vi "SaveDeviceHeader.vi"(0 "File Refnum in":refnum<file>, 1 "no. of arrays":i32, 3 "Array Lengths":i32, 5 "Filename":string, 7 "Run Number":i32, 9 "Array Titles":string, 11 "error in (no error)":errorcluster, 12 "Temperature":dbl, 13 "Humidity":dbl, 14 "Strip Segment":string) -> (4 "File Refnum out":refnum<file>, 6 "Header string":string, 10 "error out":errorcluster)   [LabVIEW 2013]
uses:
  globals/QC_RunInformation.vi
  globals/QC_MeasurementSetup.vi
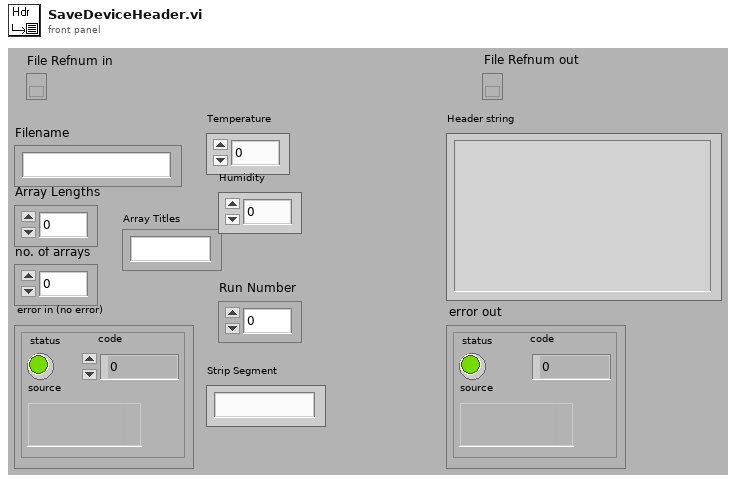
[diagram p1: front panel]
types:
  T1 = cluster{"Institute":string, "Manufacturers":string[], "Devices":string[], "Serialnumbers Lookup DB":string, "Data directory":string, "Backup & screenshot directory":string, "List of known users":string[], "Measurement switch not used":bool, "Measurement Switch":string, "DUT Switch":string, "Rseries IV [MOhm]":string, "Rshunt IV [MOhm]":string, "Rseries CV [MOhm]":string, "DC blocking Cap [µF]":string, "Rseries LCR [MOhm]":string, "Rseries stability [MOhm]":string, "Rshunt stability [MOhm]":string, "Rseries striptest bias [MOhm]":string, "Rseries strip pinhole [MOhm]":string}
  T2 = cluster{"Sensor Serial No.:":string, "Wafer:":string, "Batch:":string, "Manufacturer:":string, "Device Category:":string, "Database Serial No.:":string, "Date Initiated:":string, "Time Initiated:":string, "Test":string, "Probeplan used:":string, "End of Run comment:":string, "User:":string, "Vbias SMU":string, "LCR":string, "Test SMU":string, "Test DMM":string}
  T3 = cluster{"Supply":refnum<class "SupplyControl.lvclass">, "LCR":refnum<class "LCRControl.lvclass">, "Initial Voltage [V]":dbl, "Final Voltage [V]":dbl, "Step Size [V]":dbl, "Step Interval [s]":i32, "Number Of Steps":u32, "AC frequency [Hz]":i32, "RC Configuration":u16, "AC amplitude [V]":dbl, "Ramp down steps [V]":dbl, "Ramp down Interval [s]":i32, "Set Current Limit?":bool, "Current Limit [µA]":dbl, "Temperature Readout":enum16{"Read Arduino", "Enter manually"}, "Arduino":refnum<class "ArduinoControl.lvclass">, "Supply Name":string, "LCR Name":string, "V_depletion Limit [V]":dbl, "Switching":refnum<class "Switching.lvclass">, "Matrix used?":bool, "Matrix X Channels":cluster{"Bias Supply / SMU LO":i32, "Bias Supply / SMU HI":i32, "CV Box LO":i32, "CV Box HI":i32, "CV Box LO IN":i32, "CV Box HI IN":i32, "Volt meter LO":i32, "Volt meter HI":i32, "Mux1 C1":i32, "Mux1 C2":i32, "Mux2 C1":i32, "Mux2 C2":i32}}
  T4 = cluster{"Bias Supply":refnum<class "SupplyControl.lvclass">, "SMU":refnum<class "SupplyControl.lvclass">, "LCR":refnum<class "LCRControl.lvclass">, "Probe Card Channels":i32, "Bias Voltage [V]":dbl, "First strip":i32, "Last strip":i32, "Base Voltage [V]":dbl, "Base Ramp Step [V]":dbl, "Base Ramp Interval [ms]":u32, "High Voltage [V]":dbl, "High Ramp Step [V]":dbl, "High Ramp Interval [ms]":u32, "AC frequency [Hz]":i32, "AC amplitude [V]":dbl, "RC Configuration":u16, "Single Needle":bool, "Temperature Readout":enum16{"Read Arduino", "Enter manually"}, "Arduino":refnum<class "ArduinoControl.lvclass">, "Fraction of good strips [%]":dbl, "ProbeStation":refnum<class "ProbeStationControl.lvclass">, "Switching":refnum<class "Switching.lvclass">, "Matrix used?":bool, "Matrix X Channels":cluster{"Bias Supply / SMU LO":i32, "Bias Supply / SMU HI":i32, "CV Box LO":i32, "CV Box HI":i32, "CV Box LO IN":i32, "CV Box HI IN":i32, "Volt meter LO":i32, "Volt meter HI":i32, "Mux1 C1":i32, "Mux1 C2":i32, "Mux2 C1":i32, "Mux2 C2":i32}, "Pinholes Y/N":bool, "Capacitance Y/N":bool, "Resistance Y/N":bool, "Bias Supply Name":string, "SMU Name":string, "LCR Name":string}
  T5 = cluster{"Supply":refnum<class "SupplyControl.lvclass">, "LCR":refnum<class "LCRControl.lvclass">, "Initial Voltage [V]":dbl, "Final Voltage [V]":dbl, "Step Size [V]":dbl, "Step Interval [s]":i32, "Number Of Steps":u32, "AC frequency [Hz]":i32, "RC Configuration":u16, "AC amplitude [V]":dbl, "Ramp down steps [V]":dbl, "Ramp down Interval [s]":i32, "Set Current Limit?":bool, "Current Limit [µA]":dbl, "Temperature Readout":enum16{"Read Arduino", "Enter manually"}, "Arduino":refnum<class "ArduinoControl.lvclass">, "Supply Name":string, "LCR Name":string, "C_is Limit [pF/cm]":dbl, "Switching":refnum<class "Switching.lvclass">, "Matrix used?":bool, "Matrix X Channels":cluster{"Bias Supply / SMU LO":i32, "Bias Supply / SMU HI":i32, "CV Box LO":i32, "CV Box HI":i32, "CV Box LO IN":i32, "CV Box HI IN":i32, "Volt meter LO":i32, "Volt meter HI":i32, "Mux1 C1":i32, "Mux1 C2":i32, "Mux2 C1":i32, "Mux2 C2":i32}}
  T6 = cluster{"Supply":refnum<class "SupplyControl.lvclass">, "Voltage [V]":dbl, "Measurement Interval [s]":i32, "Test Duration":u32, "Ramp up steps [V]":dbl, "Ramp up Interval [s]":u32, "Ramp down steps [V]":dbl, "Ramp down Interval [s]":i32, "Set Current Limit?":bool, "Current Limit [µA]":dbl, "Temperature Readout":enum16{"Read Arduino", "Enter manually"}, "Arduino":refnum<class "ArduinoControl.lvclass">, "Supply Name":string, "Maximum current fluctuation [%]":dbl, "Switching.lvclass":refnum<class "Switching.lvclass">, "Matrix used?":bool, "Matrix X Channels":cluster{"Bias Supply / SMU LO":i32, "Bias Supply / SMU HI":i32, "CV Box LO":i32, "CV Box HI":i32, "CV Box LO IN":i32, "CV Box HI IN":i32, "Volt meter LO":i32, "Volt meter HI":i32, "Mux1 C1":i32, "Mux1 C2":i32, "Mux2 C1":i32, "Mux2 C2":i32}}
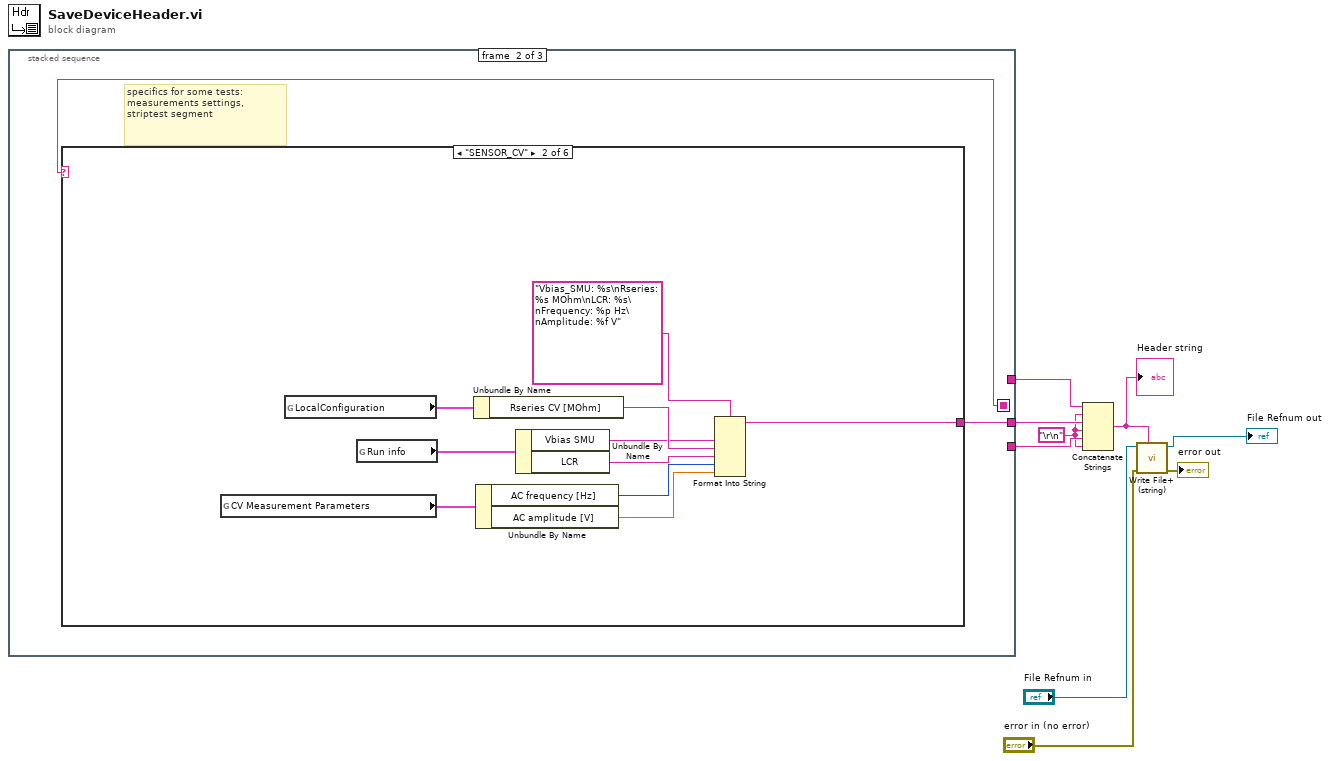
[diagram p0: block diagram]
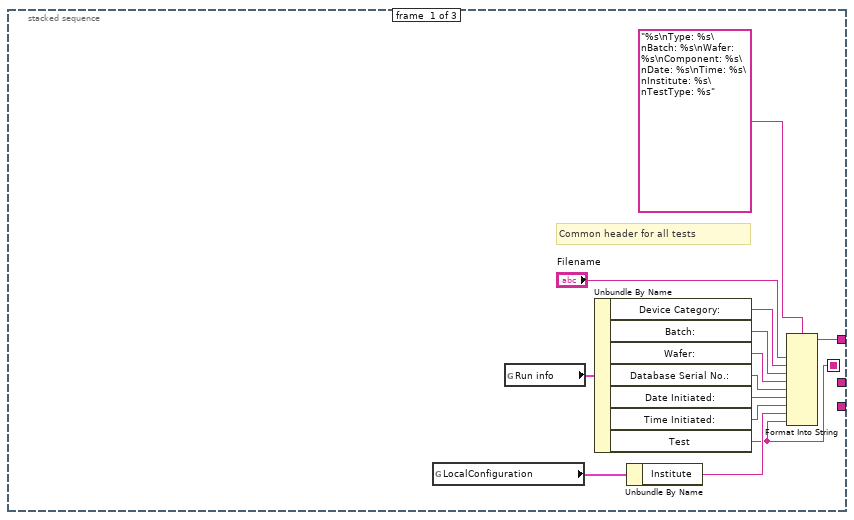
[diagram p2: hidden frame]
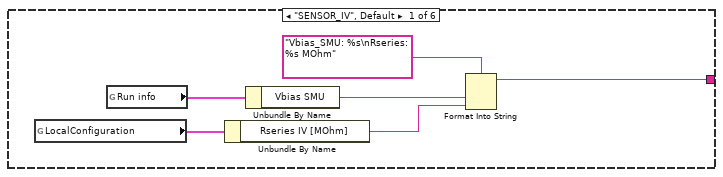
[diagram p3: hidden frame]
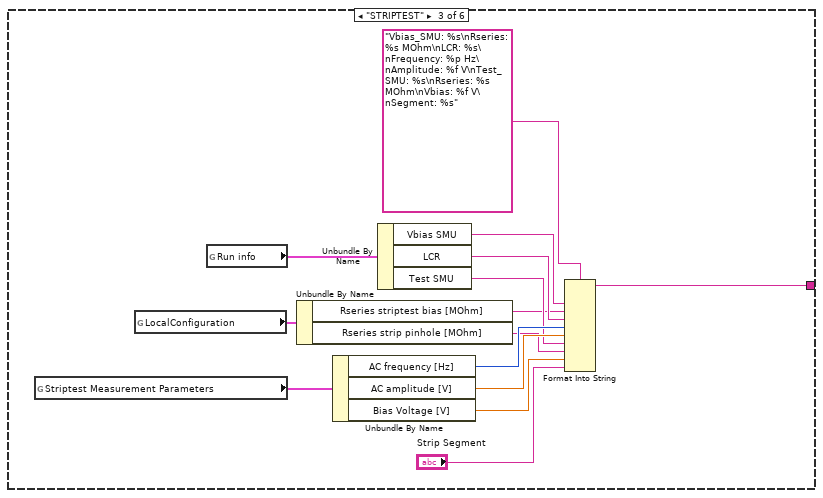
[diagram p4: hidden frame]
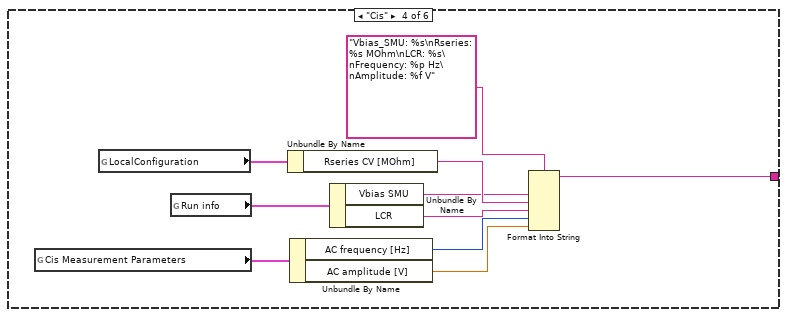
[diagram p5: hidden frame]
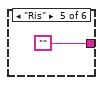
[diagram p6: hidden frame]
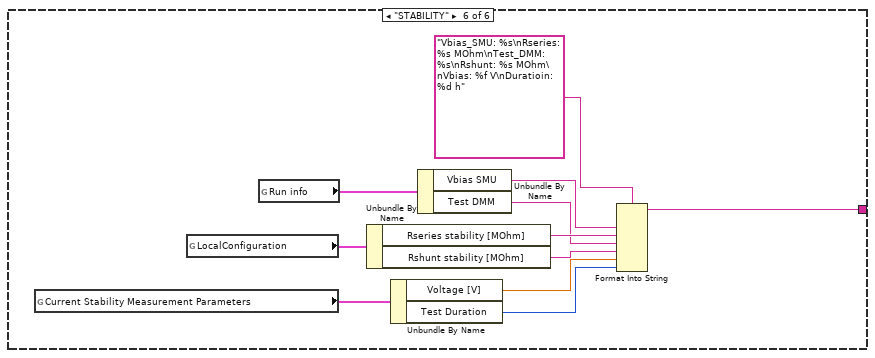
[diagram p7: hidden frame]
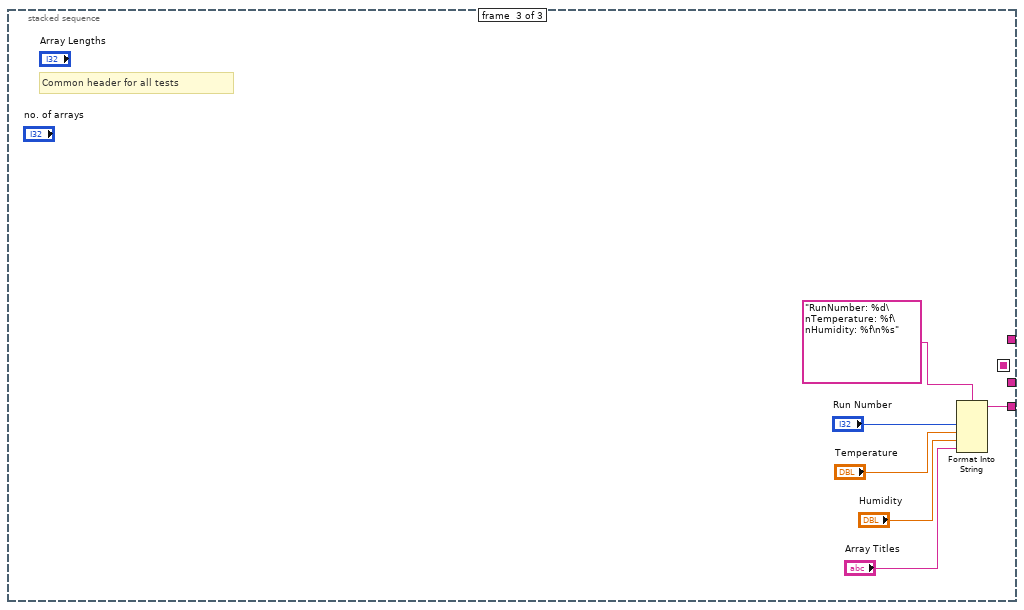
[diagram p8: hidden frame]
diagram:
  w1 = "\r\n"
  n1 = stacked-sequence {
    seq-local: [w11 _ _] -> [_ w24 _]
    tunnel: [_ w23 _] -> w5
    tunnel: [_ _ w77] -> w4
    tunnel: [w10 _ _] -> w3
    frame #0 {
      # "Common header for all tests"
      n2 = global read "QC_RunInformation.vi" "LocalConfiguration"() -> (w12:T1)
      n3 = global read "QC_RunInformation.vi" "Run info"() -> (w13:T2)
      n4 = Unbundle By Name(w13) -> ("Device Category:"=w16:string, "Batch:"=w17:string, "Wafer:"=w18:string, "Database Serial No.:"=w19:string, "Date Initiated:"=w20:string, "Time Initiated:"=w21:string, "Test"=w11:string)
      n5 = Unbundle By Name(w12) -> ("Institute"=w22:string)
      n6 = Format Into String(format string="%s\nType: %s\nBatch: %s\nWafer: %s\nComponent: %s\nDate: %s\nTime: %s\nInstitute: %s\nTestType: %s", "Filename", w16, w17, w18, w19, w20, w21, w22, w11) -> (resulting string=w10:string)  [unwired: 2 in, 1 out]
    }
    frame #1 {
      # "specifics for some tests:\nmeasurements settings,\nstriptest segment"
      n7 = case shown="\"SENSOR_CV\"" w24 {
        tunnel: [w25 w31 w51 w55 "" w72] -> w23
        frame "SENSOR_IV", Default {
          n8 = global read "QC_RunInformation.vi" "LocalConfiguration"() -> (w30:T1)
          n9 = global read "QC_RunInformation.vi" "Run info"() -> (w29:T2)
          n10 = Unbundle By Name(w30) -> ("Rseries IV [MOhm]"=w27:string)
          n11 = Unbundle By Name(w29) -> ("Vbias SMU"=w26:string)
          n12 = Format Into String(format string="Vbias_SMU: %s\nRseries: %s MOhm", w26, w27) -> (resulting string=w25:string)  [unwired: 2 in, 1 out]
        }
        frame "SENSOR_CV" {
          n13 = global read "QC_MeasurementSetup.vi" "CV Measurement Parameters"() -> (w40:T3)
          n14 = global read "QC_RunInformation.vi" "LocalConfiguration"() -> (w39:T1)
          n15 = global read "QC_RunInformation.vi" "Run info"() -> (w38:T2)
          n16 = Unbundle By Name(w39) -> ("Rseries CV [MOhm]"=w36:string)
          n17 = Unbundle By Name(w40) -> ("AC frequency [Hz]"=w33:i32, "AC amplitude [V]"=w32:dbl)
          n18 = Unbundle By Name(w38) -> ("Vbias SMU"=w35:string, "LCR"=w34:string)
          n19 = Format Into String(format string="Vbias_SMU: %s\nRseries: %s MOhm\nLCR: %s\nFrequency: %p Hz\nAmplitude: %f V", w35, w36, w34, w33, w32) -> (resulting string=w31:string)  [unwired: 2 in, 1 out]
        }
        frame "STRIPTEST" {
          n20 = global read "QC_MeasurementSetup.vi" "Striptest Measurement Parameters"() -> (w53:T4)
          n21 = global read "QC_RunInformation.vi" "LocalConfiguration"() -> (w44:T1)
          n22 = global read "QC_RunInformation.vi" "Run info"() -> (w54:T2)
          n23 = Unbundle By Name(w44) -> ("Rseries striptest bias [MOhm]"=w43:string, "Rseries strip pinhole [MOhm]"=w41:string)
          n24 = Unbundle By Name(w53) -> ("AC frequency [Hz]"=w50:i32, "AC amplitude [V]"=w49:dbl, "Bias Voltage [V]"=w42:dbl)
          n25 = Unbundle By Name(w54) -> ("Vbias SMU"=w47:string, "LCR"=w46:string, "Test SMU"=w45:string)
          n26 = Format Into String(format string="Vbias_SMU: %s\nRseries: %s MOhm\nLCR: %s\nFrequency: %p Hz\nAmplitude: %f V\nTest_SMU: %s\nRseries: %s MOhm\nVbias: %f V\nSegment: %s", w47, w43, w46, w50, w49, w45, w41, w42, "Strip Segment") -> (resulting string=w51:string)  [unwired: 2 in, 1 out]
        }
        frame "Cis" {
          n27 = global read "QC_MeasurementSetup.vi" "Cis Measurement Parameters"() -> (w64:T5)
          n28 = global read "QC_RunInformation.vi" "LocalConfiguration"() -> (w63:T1)
          n29 = global read "QC_RunInformation.vi" "Run info"() -> (w62:T2)
          n30 = Unbundle By Name(w63) -> ("Rseries CV [MOhm]"=w60:string)
          n31 = Unbundle By Name(w64) -> ("AC frequency [Hz]"=w57:i32, "AC amplitude [V]"=w56:dbl)
          n32 = Unbundle By Name(w62) -> ("Vbias SMU"=w59:string, "LCR"=w58:string)
          n33 = Format Into String(format string="Vbias_SMU: %s\nRseries: %s MOhm\nLCR: %s\nFrequency: %p Hz\nAmplitude: %f V", w59, w60, w58, w57, w56) -> (resulting string=w55:string)  [unwired: 2 in, 1 out]
        }
        frame "Ris" {
        }
        frame "STABILITY" {
          n34 = global read "QC_MeasurementSetup.vi" "Current Stability Measurement Parameters"() -> (w76:T6)
          n35 = global read "QC_RunInformation.vi" "LocalConfiguration"() -> (w75:T1)
          n36 = global read "QC_RunInformation.vi" "Run info"() -> (w74:T2)
          n37 = Unbundle By Name(w75) -> ("Rseries stability [MOhm]"=w70:string, "Rshunt stability [MOhm]"=w68:string)
          n38 = Unbundle By Name(w76) -> ("Voltage [V]"=w67:dbl, "Test Duration"=w66:u32)
          n39 = Unbundle By Name(w74) -> ("Vbias SMU"=w71:string, "Test DMM"=w69:string)
          n40 = Format Into String(format string="Vbias_SMU: %s\nRseries: %s MOhm\nTest_DMM: %s\nRshunt: %s MOhm\nVbias: %f V\nDuratioin: %d h", w71, w70, w69, w68, w67, w66) -> (resulting string=w72:string)  [unwired: 2 in, 1 out]
        }
      }
    }
    frame #2 {
      # "Common header for all tests"
      n41 = Format Into String(format string="RunNumber: %d\nTemperature: %f\nHumidity: %f\n%s", "Run Number", "Temperature", "Humidity", "Array Titles") -> (resulting string=w77:string)  [unwired: 2 in, 1 out]
    }
  }
  n42 = Concatenate Strings(w3, w1, w5, w1, w4, w1) -> (w2:string)
  "Header string" <- w2
  n43 = call <vilib>:"Write File+ (string).vi"("string"=w2, "error in (no error)"="error in (no error)", "refnum"="File Refnum in") -> ("error out"=→"error out":errorcluster, "dup refnum"=→"File Refnum out":refnum<file>)  [unwired: 4 in, 1 out]
